vi "Multiple ToFs State Machine.vi"() -> ()   [LabVIEW 2014]
uses:
  Type Defs/VL6180 states.ctl
  Type Defs/VL6180 Resource.ctl
  <vilib>/MakerHub/LINX/Public/Peripherals/Digital/Digital Write N Chans.vi
  <vilib>/MakerHub/LINX/Public/Peripherals/Digital/Digital Write 1 Chan.vi
  <vilib>/MakerHub/LINX/Public/Peripherals/Digital/Digital Read N Chans.vi
  <vilib>/MakerHub/LINX/Public/Peripherals/Analog/Analog Read N Chans.vi
  <vilib>/MakerHub/LINX/Private/Local IO/LinxDigitalWrite.vi
  <vilib>/MakerHub/LINX/Public/Utilities/Check Channel.vi
  <vilib>/MakerHub/LINX/Private/Local IO/LinxDigitalRead.vi
  <vilib>/MakerHub/LINX/Private/Local IO/LinxAnalogRead.vi
  <vilib>/myRIO/Instrument Drivers/Onboard IO/DIO/vis/Write.vi
  <vilib>/MakerHub/LINX/Private/myRIO/Utilities/Get DIO Channel Name.vi
  <vilib>/myRIO/Instrument Drivers/Onboard IO/DIO/vis/Read.vi
  <vilib>/myRIO/Instrument Drivers/Onboard IO/AI/vis/Read.vi
  <vilib>/MakerHub/LINX/Public/Utilities/Open Local.vi
  <vilib>/MakerHub/LINX/Private/Utilties/Generate Error.vi
  <vilib>/myRIO/Instrument Drivers/Onboard IO/DIO/vis/Smart Open.vi
  <vilib>/Utility/error.llb/Error Cluster From Error Code.vi
  <vilib>/myRIO/Common/Instrument Driver Framework/myRIO v1.0/DIO/vis/myRIO v1.0 Write DIO.vi
  <vilib>/myRIO/Common/Instrument Driver Framework/myRIO v1.0/DIO/vis/myRIO v1.0 Read DIO.vi
  <vilib>/MakerHub/LINX/Private/myRIO/Utilities/Get AI Channel Name.vi
  <vilib>/myRIO/Instrument Drivers/Onboard IO/AI/vis/Smart Open.vi
  <vilib>/myRIO/Common/Instrument Driver Framework/myRIO v1.0/AI/vis/myRIO v1.0 Read AI.vi
  <vilib>/MakerHub/LINX/LMH-LINX.lvlib
panel:
  out "Current":dbl(knob) scale=0.0..12.0
  out "Voltage":dbl(knob) scale=0.0..12.0
  out "Track Position Sensor 2":bool
  out "Track Position Sensor 1":bool
  in  "# of sensors":i32=3
  out "ToF 7":u8(slide) scale=0.0..80.0
  out "ToF 6":u8(slide) scale=0.0..80.0
  out "ToF 5":u8(slide) scale=0.0..80.0
  out "Sensors Online":bool[](array[boolean])
  out "Status":string
  in  "I2C Channel":u8
  out "ToF 4":u8(slide) scale=0.0..80.0
  out "ToF 3":u8(slide) scale=0.0..80.0
  out "ToF 2":u8(slide) scale=0.0..80.0
  out "Sensor Error Code":u8
  out "Attempts":i32
  out "ToF 1":u8(slide) scale=0.0..80.0
  out "error out":errorcluster
  in  "Speed Read":bool
  out "Loop Rate (Hz)":u32
  in  "milliseconds to wait":u32=5
  in  "Stop":bool
  # "0 = No error\n6 = early convergence estimate check failed\n7 = max convergence issue"
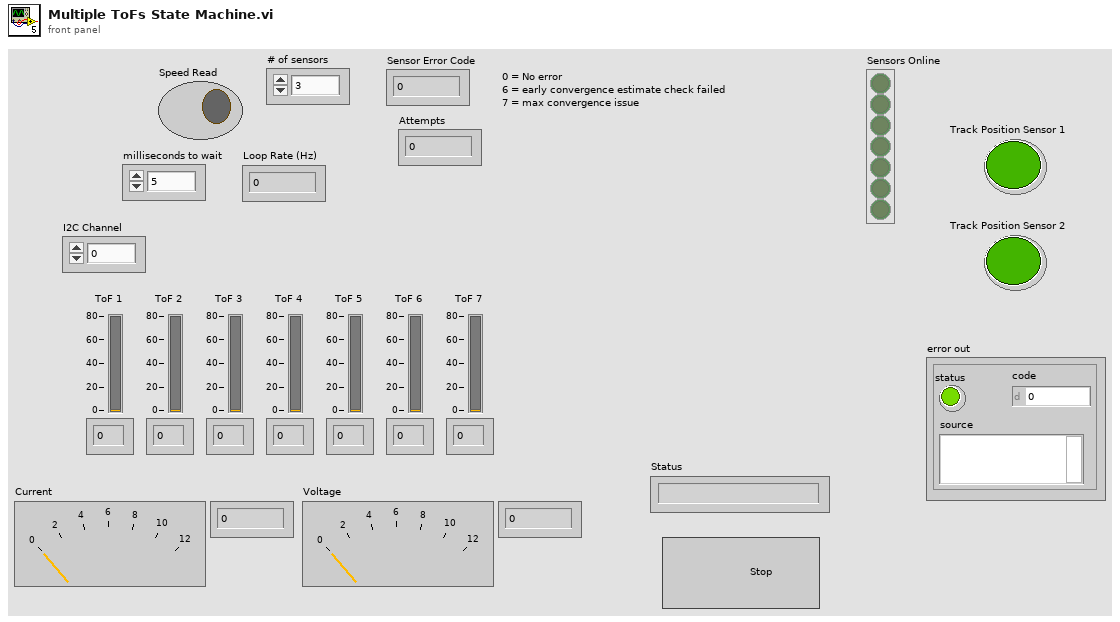
[diagram p1: front panel]
types:
  T1 = typedef "VL6180 states.ctl" = enum16{"Ping All", "Initialize", "Read"}
  T2 = typedef "LMH-LINX.lvlib/LINX Ref.ctl" = cluster{"IO":T3, "Interface":T4, "LINX Device Config":T5}
  T3 = typedef "LMH-LINX.lvlib/Platform.ctl" = enum16{"Remote", "Local"}
  T4 = typedef "LMH-LINX.lvlib/Interface.ctl" = enum16{"Serial", "TCP"}
  T5 = typedef "LMH-LINX.lvlib/Device.lvlib/LINX Device Config.ctl" = cluster{"Interface":T4, "COM Port":refnum<visa-resource-name>, "TCP Configuration":T6, "Device Family":u8, "Device ID":u8, "Device Name":string, "TCP Ref":refnum<k5>, "Channels":T7}
  T6 = typedef "LMH-LINX.lvlib/Device.lvlib/TCP Config.ctl" = cluster{"IP Address":string, "Port":u16}
  T7 = typedef "LMH-LINX.lvlib/Channels.ctl" = cluster{"DI":u8[], "DO":u8[], "AI":u8[], "AO":u8[], "PWM":u8[], "QE":u8[], "UART":u8[], "I2C 2":u8[], "SPI":u8[], "CAN":u8[], "Servo":u8[], "AI Ref (V)":dbl, "AI Resolution (Bits)":u8, "AO Ref (V)":dbl, "AO Resolution (Bits)":u8}
  T8 = typedef "VL6180 Resource.ctl" = cluster{"I2C Channel":u8, "I2C Slave Address":u8, "Online":bool}
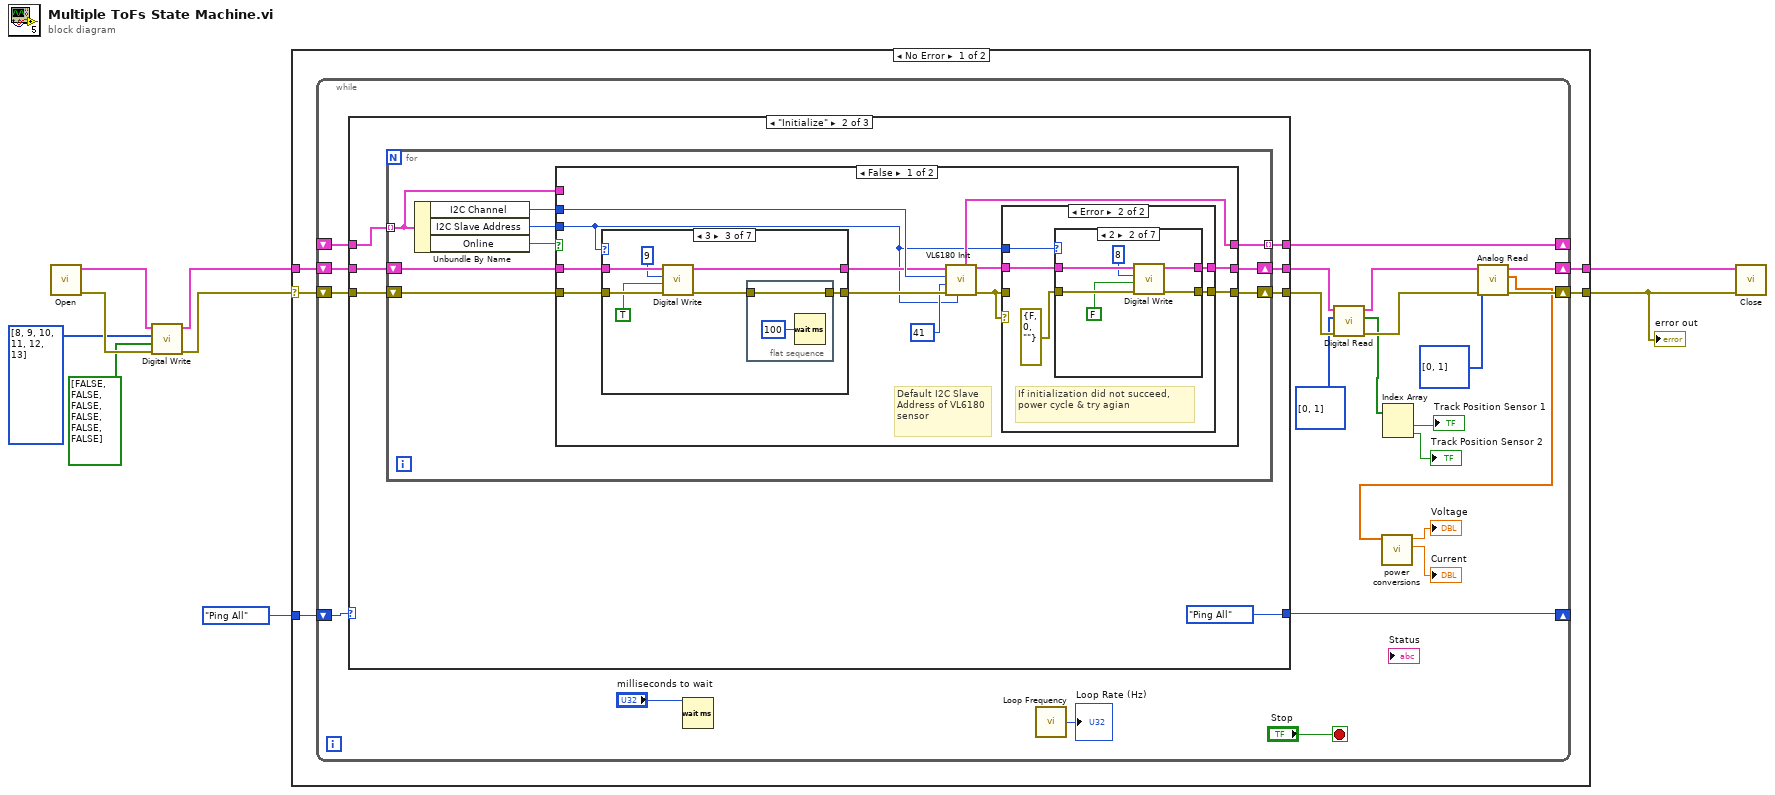
[diagram p0: block diagram]
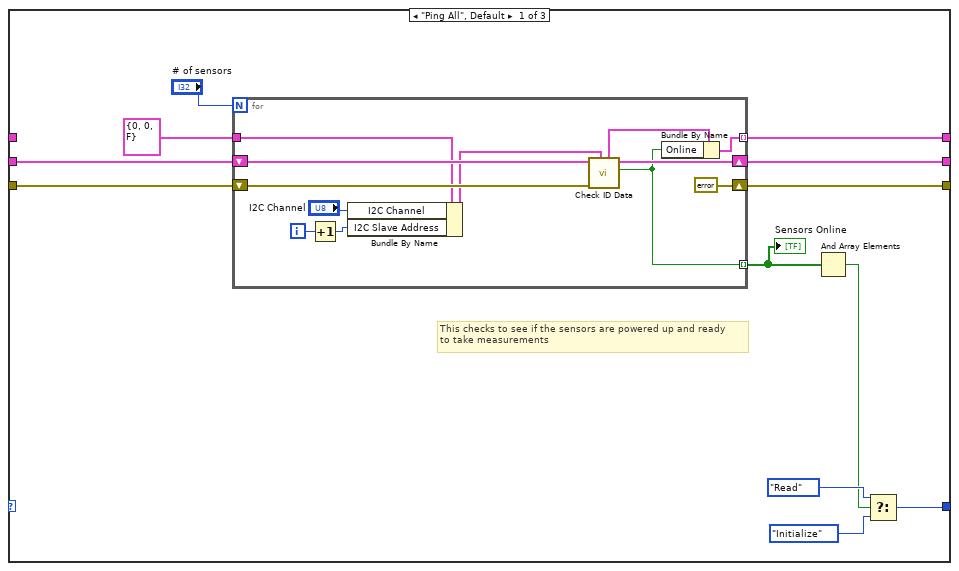
[diagram p2: hidden frame]
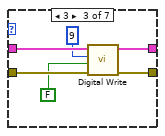
[diagram p5: hidden frame]
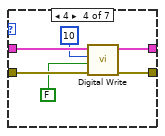
[diagram p6: hidden frame]
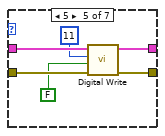
[diagram p7: hidden frame]
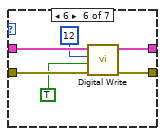
[diagram p8: hidden frame]
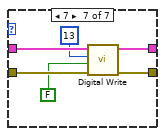
[diagram p9: hidden frame]
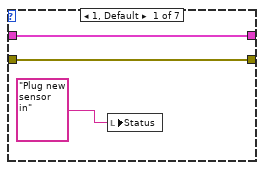
[diagram p10: hidden frame]
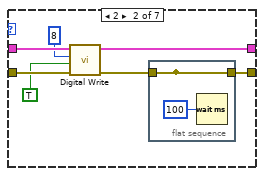
[diagram p11: hidden frame]
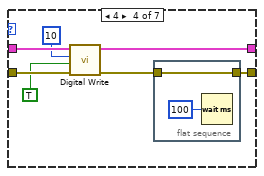
[diagram p12: hidden frame]
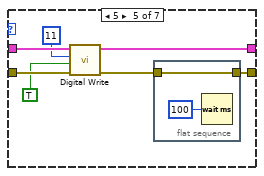
[diagram p13: hidden frame]
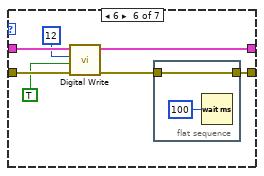
[diagram p14: hidden frame]
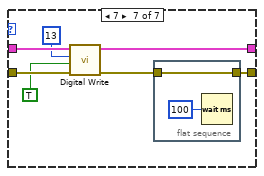
[diagram p15: hidden frame]
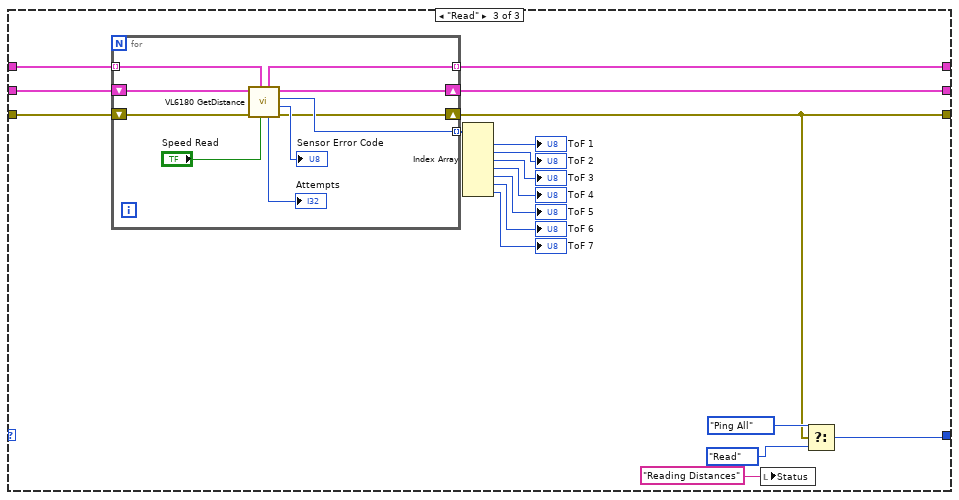
[diagram p17: hidden frame]
diagram:
  n1 = call-poly <vilib>:"Open.vi"() -> ("Error Out"=w6:errorcluster, "LINX Resource"=w3:T2)  [unwired: 9 in, 1 out]
  n2 = call-poly <vilib>:"Digital Write.vi"("Error In"=w6, "Values"=bool[] [FALSE, FALSE, FALSE, FALSE, FALSE, FALSE], "DO Channels"=u8[] [8, 9, 10, 11, 12, 13], "LINX Resource"=w3) -> ("Error Out"=w1:errorcluster, "LINX Resource"=w2:T2)  [unwired: 6 in]
  n3 = case shown="No Error" w1 {
    selector: w1 -> [w12 w224]
    tunnel: [w14 w224] -> w9
    tunnel: [w13 w223] -> w7
    tunnel: VL6180_states."Ping All" -> [w11 _]
    tunnel: w2 -> [w10 w223]
    frame No Error {
      n4 = while {
        shift-right: [w27] -> w13
        shift-left: w10 -> [w34]
        shift-right: [w26] -> w14
        shift-left: w12 -> [w33]
        shift-right: [w31] -> _
        shift-left: _ -> [w32]
        shift-right: [w29] -> _
        shift-left: w11 -> [w30]
        stop <- "Stop" stop-if-true
        n5 = case shown="\"Initialize\"" w30 {
          tunnel: w34 -> [w49 w68 w210]
          tunnel: w33 -> [w48 w62 w212]
          tunnel: w32 -> [_ w66 w209]
          tunnel: [w46 w63 w211] -> w31
          tunnel: [w47 w65 w195] -> w25
          tunnel: [w41 VL6180_states."Ping All" w203] -> w29
          tunnel: [w40 w64 w196] -> w24
          frame "Ping All", Default {
            # "This checks to see if the sensors are powered up and ready\nto take measurements"
            n6 = for {
              N: "# of sensors" -> [_]
              tunnel: T8 {"I2C Channel"=0, "I2C Slave Address"=0, "Online"=FALSE} ("VL6180 Resource out") -> [w54]
              shift-right: [w57] -> w47
              shift-left: w49 -> [w61]
              tunnel: [w56] -> w46 mode=indexing
              tunnel: [w55] -> w45 mode=indexing
              shift-right: [errorcluster {"status"=FALSE, "code"=0, "source"=""} ("error IO")] -> w40
              shift-left: w48 -> [w60]
              i -> [w58]
              n7 = Increment(x=w58) -> (x+1=w51:i32)
              n8 = Bundle By Name(cluster=w54, "I2C Channel"="I2C Channel", "I2C Slave Address"=w51) -> (w53:T8)
              n9 = call "Check ID Data.vi"("VL6180 Resource"=w53, "Error In"=w60, "LINX Resource"=w61) -> ("Same Model?"=w55:bool, "LINX Resource"=w57:T2, "VL6180 Resource"=w59:T8)  [unwired: 5 in, 1 out]
              n10 = Bundle By Name(cluster=w59, "Online"=w55) -> (w56:T8)
            }
            "Sensors Online" <- w45
            n11 = And Array Elements(Boolean array=w45) -> (logical AND=w42:bool)
            n12 = Select(t=VL6180_states."Read", s=w42, f=VL6180_states."Initialize") -> (s? t:f=w41:T1)
          }
          frame "Initialize" {
            n13 = for {
              tunnel: w66 -> [w71] mode=indexing
              shift-right: [w75] -> w65
              shift-left: w68 -> [w77]
              shift-right: [w74] -> w64
              shift-left: w62 -> [w69]
              tunnel: [w70] -> w63 mode=indexing
              n14 = Unbundle By Name(w71) -> ("I2C Channel"=w73:u8, "I2C Slave Address"=w72:u8, "Online"=w76:bool)
              n15 = case shown="False" w76 {
                tunnel: w77 -> [w88 w194]
                tunnel: w69 -> [w85 w193]
                tunnel: [w82 w194] -> w75
                tunnel: [w81 w193] -> w74
                tunnel: w73 -> [w89 _]
                tunnel: w72 -> [w79 _]
                tunnel: w71 -> [_ w192]
                tunnel: [w83 w192] -> w70
                frame False {
                  # "Default I2C Slave Address of VL6180 sensor"
                  n16 = case shown="3" w79 {
                    tunnel: w88 -> [w136 w144 w153 w162 w171 w180 w189]
                    tunnel: [w136 w143 w152 w161 w170 w179 w188] -> w87
                    tunnel: [w135 w139 w147 w156 w165 w174 w183] -> w86
                    tunnel: w85 -> [w135 w142 w151 w160 w169 w178 w187]
                    frame 1, Default {
                      n17 = local write "Status"("Plug new sensor in" ("message")) -> ()
                    }
                    frame 2 {
                      n18 = call-poly <vilib>:"Digital Write.vi"("Error In"=w142, "Output Value"=TRUE, "DO Channel"=u8 8, "LINX Resource"=w144) -> ("Error Out"=w138:errorcluster, "LINX Resource"=w143:T2)  [unwired: 6 in]
                      n19 = flat-sequence {
                        tunnel: [w145] -> _
                        tunnel: [w145] -> w139
                        tunnel: w138 -> [w145]
                        frame #0 {
                          n20 = Wait (ms)(milliseconds to wait=u32 100) -> ()  [unwired: 1 out]
                        }
                      }
                    }
                    frame 3 {
                      n21 = call-poly <vilib>:"Digital Write.vi"("Error In"=w151, "Output Value"=TRUE, "DO Channel"=u8 9, "LINX Resource"=w153) -> ("Error Out"=w148:errorcluster, "LINX Resource"=w152:T2)  [unwired: 6 in]
                      n22 = flat-sequence {
                        tunnel: w148 -> [w154]
                        tunnel: [w154] -> w147
                        frame #0 {
                          n23 = Wait (ms)(milliseconds to wait=u32 100) -> ()  [unwired: 1 out]
                        }
                      }
                    }
                    frame 4 {
                      n24 = call-poly <vilib>:"Digital Write.vi"("Error In"=w160, "Output Value"=TRUE, "DO Channel"=u8 10, "LINX Resource"=w162) -> ("Error Out"=w157:errorcluster, "LINX Resource"=w161:T2)  [unwired: 6 in]
                      n25 = flat-sequence {
                        tunnel: w157 -> [w163]
                        tunnel: [w163] -> w156
                        frame #0 {
                          n26 = Wait (ms)(milliseconds to wait=u32 100) -> ()  [unwired: 1 out]
                        }
                      }
                    }
                    frame 5 {
                      n27 = call-poly <vilib>:"Digital Write.vi"("Error In"=w169, "Output Value"=TRUE, "DO Channel"=u8 11, "LINX Resource"=w171) -> ("Error Out"=w166:errorcluster, "LINX Resource"=w170:T2)  [unwired: 6 in]
                      n28 = flat-sequence {
                        tunnel: w166 -> [w172]
                        tunnel: [w172] -> w165
                        frame #0 {
                          n29 = Wait (ms)(milliseconds to wait=u32 100) -> ()  [unwired: 1 out]
                        }
                      }
                    }
                    frame 6 {
                      n30 = call-poly <vilib>:"Digital Write.vi"("Error In"=w178, "Output Value"=TRUE, "DO Channel"=u8 12, "LINX Resource"=w180) -> ("Error Out"=w175:errorcluster, "LINX Resource"=w179:T2)  [unwired: 6 in]
                      n31 = flat-sequence {
                        tunnel: w175 -> [w181]
                        tunnel: [w181] -> w174
                        frame #0 {
                          n32 = Wait (ms)(milliseconds to wait=u32 100) -> ()  [unwired: 1 out]
                        }
                      }
                    }
                    frame 7 {
                      n33 = call-poly <vilib>:"Digital Write.vi"("Error In"=w187, "Output Value"=TRUE, "DO Channel"=u8 13, "LINX Resource"=w189) -> ("Error Out"=w184:errorcluster, "LINX Resource"=w188:T2)  [unwired: 6 in]
                      n34 = flat-sequence {
                        tunnel: w184 -> [w190]
                        tunnel: [w190] -> w183
                        frame #0 {
                          n35 = Wait (ms)(milliseconds to wait=u32 100) -> ()  [unwired: 1 out]
                        }
                      }
                    }
                  }
                  n36 = call "VL6180 Init.vi"("Change Slave Address"=w79, "Error In"=w86, "I2C Slave Address (0)"=u8 41, "I2C Channel"=w89, "LINX Resource"=w87) -> ("Error Out"=w78:errorcluster, "LINX Resource"=w80:T2, "VL6180 Resource"=w83:T8)  [unwired: 4 in]
                  n37 = case shown="Error" w78 {
                    tunnel: [w91 w96] -> w82
                    tunnel: [w90 w95] -> w81
                    tunnel: w80 -> [w91 w94]
                    tunnel: w78 -> [w90 _]
                    tunnel: w79 -> [_ w93]
                    frame No Error {
                      # "Initialization successful"
                    }
                    frame Error {
                      # "If initialization did not succeed, power cycle & try agian"
                      n38 = case shown="2" w93 {
                        tunnel: w94 -> [w98 w104 w110 w116 w122 w128 w134]
                        tunnel: [w98 w103 w109 w115 w121 w127 w133] -> w96
                        tunnel: [w97 w102 w108 w114 w120 w126 w132] -> w95
                        tunnel: errorcluster {"status"=FALSE, "code"=0, "source"=""} ("Error Out") -> [w97 w101 w107 w113 w119 w125 w131]
                        frame 1, Default {
                        }
                        frame 2 {
                          n39 = call-poly <vilib>:"Digital Write.vi"("Error In"=w101, "Output Value"=FALSE, "DO Channel"=u8 8, "LINX Resource"=w104) -> ("Error Out"=w102:errorcluster, "LINX Resource"=w103:T2)  [unwired: 6 in]
                        }
                        frame 3 {
                          n40 = call-poly <vilib>:"Digital Write.vi"("Error In"=w107, "Output Value"=FALSE, "DO Channel"=u8 9, "LINX Resource"=w110) -> ("Error Out"=w108:errorcluster, "LINX Resource"=w109:T2)  [unwired: 6 in]
                        }
                        frame 4 {
                          n41 = call-poly <vilib>:"Digital Write.vi"("Error In"=w113, "Output Value"=FALSE, "DO Channel"=u8 10, "LINX Resource"=w116) -> ("Error Out"=w114:errorcluster, "LINX Resource"=w115:T2)  [unwired: 6 in]
                        }
                        frame 5 {
                          n42 = call-poly <vilib>:"Digital Write.vi"("Error In"=w119, "Output Value"=FALSE, "DO Channel"=u8 11, "LINX Resource"=w122) -> ("Error Out"=w120:errorcluster, "LINX Resource"=w121:T2)  [unwired: 6 in]
                        }
                        frame 6 {
                          n43 = call-poly <vilib>:"Digital Write.vi"("Error In"=w125, "Output Value"=TRUE, "DO Channel"=u8 12, "LINX Resource"=w128) -> ("Error Out"=w126:errorcluster, "LINX Resource"=w127:T2)  [unwired: 6 in]
                        }
                        frame 7 {
                          n44 = call-poly <vilib>:"Digital Write.vi"("Error In"=w131, "Output Value"=FALSE, "DO Channel"=u8 13, "LINX Resource"=w134) -> ("Error Out"=w132:errorcluster, "LINX Resource"=w133:T2)  [unwired: 6 in]
                        }
                      }
                    }
                  }
                }
                frame True {
                }
              }
            }
          }
          frame "Read" {
            n45 = for {
              tunnel: [w218] -> w211 mode=indexing
              shift-right: [w216] -> w195
              shift-left: w210 -> [w217]
              tunnel: w209 -> [w215] mode=indexing
              tunnel: [w214] -> w208 mode=indexing
              shift-right: [w213] -> w196
              shift-left: w212 -> [w222]
              n46 = call "VL6180 GetDistance.vi"("Speed Read"="Speed Read", "VL6180 Resource in"=w215, "error in (no error)"=w222, "LINX Resource"=w217) -> ("error out"=w213:errorcluster, "Sensor Error Code"=→"Sensor Error Code":u8, "Distance (mm)"=w214:u8, "LINX Resource"=w216:T2, "Attempts"=→"Attempts":i32, "VL6180 Resource out"=w218:T8)  [unwired: 2 in]
            }
            n47 = Index Array(array=w208) -> (element #1=→"ToF 1":u8, element #2=→"ToF 2":u8, element #3=→"ToF 3":u8, element #4=→"ToF 4":u8, element #5=→"ToF 5":u8, element #6=→"ToF 6":u8, element #7=→"ToF 7":u8)  [unwired: 7 in]
            n48 = local write "Status"("Reading Distances" ("Status")) -> ()
            n49 = Select(t=VL6180_states."Ping All", s=w196, f=VL6180_states."Read") -> (s? t:f=w203:T1)
          }
        }
        n50 = Wait (ms)(milliseconds to wait="milliseconds to wait") -> ()  [unwired: 1 out]
        n51 = call <vilib>:"Loop Frequency.vi"() -> ("Loop Rate (Hz)"=→"Loop Rate (Hz)":u32)
        n52 = call-poly <vilib>:"Digital Read.vi"("Error In"=w24, "DI Channels"=u8[] [0, 1] ("AI Channel(s)"), "LINX Resource"=w25) -> ("Error Out"=w22:errorcluster, "Values"=w20:bool[], "LINX Resource"=w23:T2)  [unwired: 6 in]
        n53 = Index Array(array=w20) -> (element #1=→"Track Position Sensor 1":bool, element #2=→"Track Position Sensor 2":bool)  [unwired: 2 in]
        n54 = call-poly <vilib>:"Analog Read.vi"("Error In"=w22, "AI Channel(s)"=u8[] [0, 1], "LINX Resource"=w23) -> ("Error Out"=w26:errorcluster, "Voltages"=w17:dbl[], "LINX Resource"=w27:T2)  [unwired: 5 in, 1 out]
        n55 = call "power conversions.vi"("Voltages"=w17) -> ("Current"=→"Current":dbl, "Voltage"=→"Voltage":dbl)  [unwired: 9 in]
      }
    }
    frame Error {
    }
  }
  "error out" <- w9
  n56 = call <vilib>:"Close.vi"("Error In"=w9, "LINX Resource"=w7) -> ()  [unwired: 9 in, 1 out]
